vi "SetPin.vi"(0 "NXP LPCXpresso54608 in":refnum<class "NXP LPCXpresso54608.lvclass">, 5 "Port":u8, 7 "Pin":u8, 9 "Value":bool, 11 "error in (no error)":errorcluster) -> (4 "NXP LPCXpresso54608 out":refnum<class "NXP LPCXpresso54608.lvclass">, 15 "error out":errorcluster)   [LabVIEW 2020, in "NXP LPCXpresso54608.lvclass"]
doc: "Sends a command to write on a pin of the target device."
uses:
  NXP LPCXpresso54608.lvclass
  Controls/Device Command Code.ctl
  Controls/Device Code.ctl
  NXP LPCXpresso54608.lvclass/NXP LPCXpresso54608.ctl
  595ea04d-fbb6-4feb-90a4-72aa54be3cc8.vi
  Read Serial Port.vi
  Write Serial Port.vi
  <vilib>/Utility/error.llb/Error Cluster From Error Code.vi
  <vilib>/ErrorRing/Error Ring.xnode
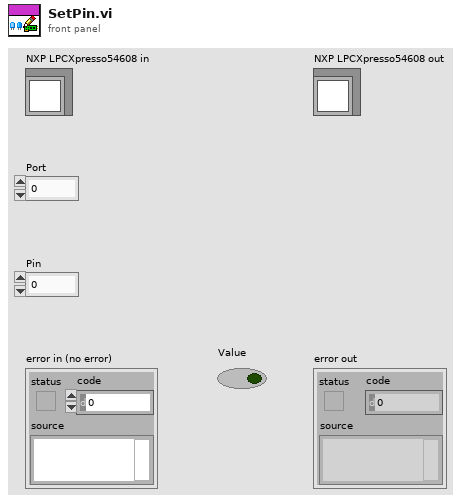
[diagram p1: front panel]
types:
  T1 = typedef "Device Code.ctl" = string
  T2 = typedef "Device Command Code.ctl" = string
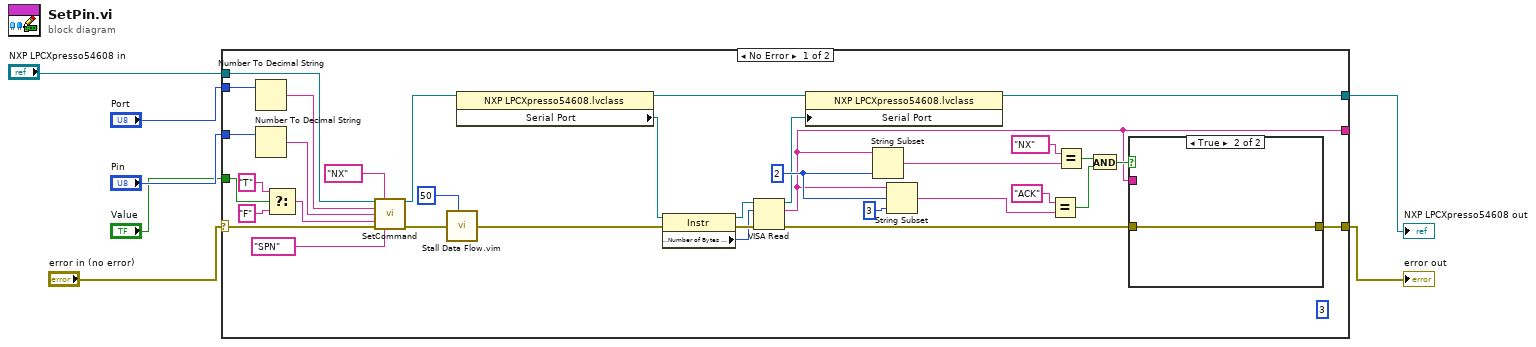
[diagram p0: block diagram]
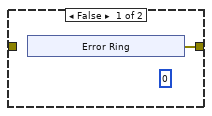
[diagram p2: hidden frame]
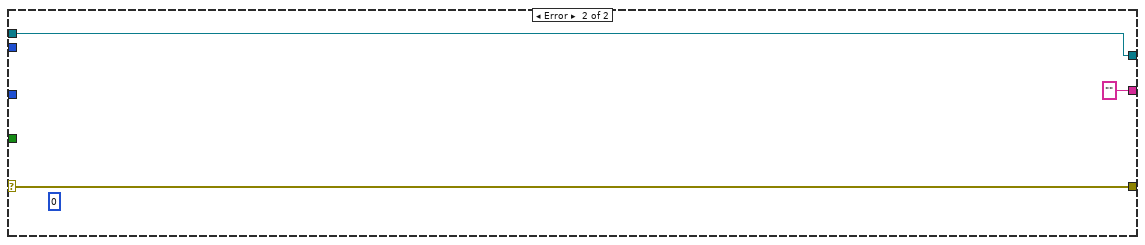
[diagram p3: hidden frame]
diagram:
  n1 = case shown="No Error" "error in (no error)" {
    selector: "error in (no error)" -> [w42 w51]
    tunnel: [w25 w51] -> w1
    tunnel: "NXP LPCXpresso54608 in" -> [w40 w52]
    tunnel: [w21 w52] -> w2
    tunnel: "Port" -> [w38 _]
    tunnel: [w15 "" ("read buffer")] -> _
    tunnel: "Pin" -> [w14 _]
    tunnel: "Value" -> [w12 _]
    frame No Error {
      (unwired) 3 ("length (rest)")
      w30 = 2 ("length (rest)")
      n2 = Number To Decimal String(number=w38) -> (decimal integer string=w37:string)  [unwired: 1 in]
      n3 = Number To Decimal String(number=w14) -> (decimal integer string=w13:string)  [unwired: 1 in]
      n4 = Select(t="T", s=w12, f="F") -> (s? t:f=w9:string)
      n5 = call-dynamic "SetCommand.vi"("NXP LPCXpresso54608 in"=w40, "Device Code"=T1 "NX", "Parameter 1"=w37, "Parameter 2"=w13, "Parameter 3"=w9, "error in (no error)"=w42, "Command Code"=T2 "SPN") -> ("NXP LPCXpresso54608 out"=w36:refnum<class "NXP LPCXpresso54608.lvclass">, "error out"=w18:errorcluster)  [unwired: 6 in, 1 out]
      n6 = call "Stall Data Flow.vim"("value in"=w18, "milliseconds to wait"=u32 50) -> ("value out"=w17:errorcluster)  [unwired: 1 out]
      n7 = property class="NXP LPCXpresso54608.lvclass"(reference=w36) -> (reference out=w22:refnum<class "NXP LPCXpresso54608.lvclass">, "Serial Port"=w35:refnum<visa-resource-name>)  [unwired: 1 in, 1 out]
      n8 = property class="Instr"(reference=w35, error in=w17) -> (reference out=w33:refnum<visa-resource-name>, error out=w34:errorcluster, "Serial Settings:Number of Bytes at Serial Port"=w32:u32)
      n9 = VISA Read(VISA resource name=w33, byte count=w32, error in (no error)=w34) -> (VISA resource name out=w20:refnum<visa-resource-name>, read buffer=w15:string, error out=w26:errorcluster)  [unwired: 1 out]
      n10 = property class="NXP LPCXpresso54608.lvclass"(reference=w22, "Serial Port"=w20) -> (reference out=w21:refnum<class "NXP LPCXpresso54608.lvclass">)  [unwired: 1 in, 1 out]
      n11 = String Subset(string=w15, length (rest)=w30) -> (substring=w23:string)  [unwired: 1 in]
      n12 = String Subset(string=w15, offset (0)=w30, length (rest)=3 ("length (rest)")) -> (substring=w31:string)
      n13 = Equal?(x="ACK", y=w31) -> (x = y?=w28:bool)
      n14 = Equal?(x=T1 "NX" ("Device Code"), y=w23) -> (x = y?=w24:bool)
      n15 = And(x=w24, y=w28) -> (x .and. y?=w27:bool)
      n16 = case shown="True" w27 {
        tunnel: w26 -> [_ w49]
        tunnel: [w43 w49] -> w25
        tunnel: w15 -> [_ _]
        frame False {
          (unwired) u8 0
          n17 = xnode "Error Ring"() -> ("error out"=w43:errorcluster)
        }
        frame True {
        }
      }
    }
    frame Error {
      (unwired) u8 0
    }
  }
  "error out" <- w1
  "NXP LPCXpresso54608 out" <- w2
